vi "Initialize Waveform UI.vi"(8 "error in":errorcluster, 10 "Waveforms UI Ctrl Ref":T2, 11 "Waveform Meas Config Ctrl Ref":T1) -> (0 "error out":errorcluster)   [LabVIEW 2025, in "Fgen Script Mode UI.lvlib"]
uses:
  Fgen Script Mode UI.lvlib
  Typedef/Waveforms UI Ctrl Ref.ctl
  Typedef/Waveform Meas Config Ctrl Ref.ctl
  Typedef/Wfm Typedef.ctl
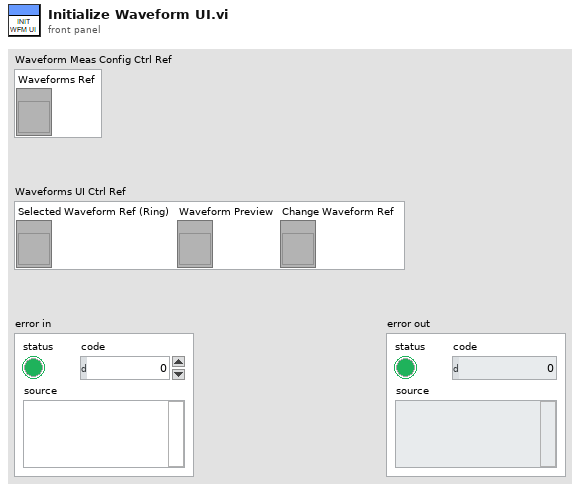
[diagram p1: front panel]
types:
  T1 = typedef "Fgen Script Mode UI.lvlib/Waveform Meas Config Ctrl Ref.ctl" = cluster{"Waveforms Ref":refnum<vi>}
  T2 = typedef "Fgen Script Mode UI.lvlib/Waveforms UI Ctrl Ref.ctl" = cluster{"Selected Waveform Ref (Ring)":refnum<vi>, "Waveform Preview":refnum<vi>, "Change Waveform Ref":refnum<vi>}
  T3 = typedef "Fgen Script Mode UI.lvlib/Wfm Typedef.ctl" = cluster{"Name":string, "Path":string, "Grp":string, "Chn":string}
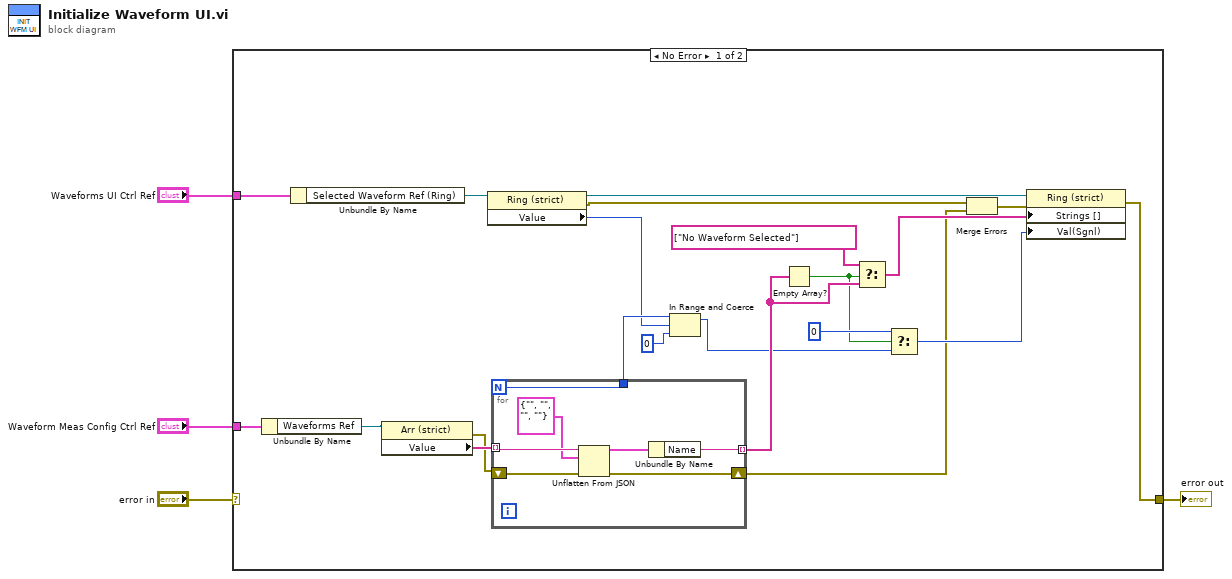
[diagram p0: block diagram]
diagram:
  n1 = case shown="No Error" "error in" {
    selector: "error in" -> [_ w33]
    tunnel: [w16 w33] -> w3
    tunnel: "Waveform Meas Config Ctrl Ref" -> [w19 _]
    tunnel: "Waveforms UI Ctrl Ref" -> [w25 _]
    frame No Error {
      n2 = Unbundle By Name(w19) -> ("Waveforms Ref"=w23:refnum<vi>)
      n3 = Unbundle By Name(w25) -> ("Selected Waveform Ref (Ring)"=w24:refnum<vi>)
      n4 = property class="Arr (strict)"(reference=w23) -> (error out=w15:errorcluster, "Value"=w18:string[])  [unwired: 1 in, 1 out]
      n5 = property class="Ring (strict)"(reference=w24) -> (reference out=w14:refnum<vi>, error out=w5:errorcluster, "Value"=w10:u16)  [unwired: 1 in]
      n6 = for {
        N -> [w26]
        tunnel: w18 -> [w32] mode=indexing
        tunnel: [w29] -> w17 mode=indexing
        shift-right: [w28] -> w6
        shift-left: w15 -> [w27]
        tunnel: [w26] -> w11
        n7 = Unflatten From JSON(JSON string=w32, type and defaults=T3 {"Name"="", "Path"="", "Grp"="", "Chn"=""} ("Waveform"), error in (no error)=w27) -> (value=w30:T3, error out=w28:errorcluster)  [unwired: 4 in]
        n8 = Unbundle By Name(w30) -> ("Name"=w29:string)
      }
      n9 = In Range and Coerce(upper limit=w11, x=w10, lower limit=0) -> (coerced(x)=w8:i32)  [unwired: 1 out]
      n10 = Empty Array?(array=w17) -> (empty?=w12:bool)
      n11 = Select(t=string[] ["No Waveform Selected"] ("Strings []"), s=w12, f=w17) -> (s? t:f=w21:string[])
      n12 = Select(t=u16 0 ("Value"), s=w12, f=w8) -> (s? t:f=w13:i32)
      n13 = Merge Errors(w5, w6) -> (w7:errorcluster)
      n14 = property class="Ring (strict)"(reference=w14, error in=w7, "Strings []"=w21, "Val(Sgnl)"=w13) -> (error out=w16:errorcluster)  [unwired: 1 out]
    }
    frame Error {
    }
  }
  "error out" <- w3
